vi "FiberSpectrograph_issueCommand_start.vi"(8 "error in (no error)":errorcluster, 11 "command_start_Ctl":T1) -> (0 "error out":errorcluster, 2 "function return":i32, 3 "command_start_Ctl out":T1)   [LabVIEW 2016, in "SALLV_FiberSpectrograph.lvlib"]
doc: "int FiberSpectrograph_shm_issueCommand_startLV(FiberSpectrograph_command_startLV *command_start_Ctl );"
uses:
  SALLV_FiberSpectrograph.lvlib
  DataTypes/command_start.ctl
  SALLV_FiberSpectrograph.so
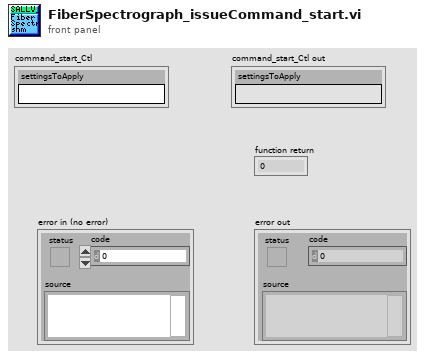
[diagram p1: front panel]
types:
  T1 = typedef "SALLV_FiberSpectrograph.lvlib/command_start.ctl" = cluster{"settingsToApply":string}
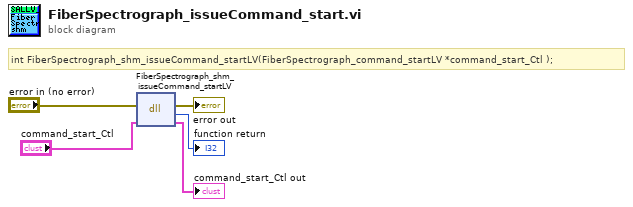
[diagram p0: block diagram]
diagram:
  # "int FiberSpectrograph_shm_issueCommand_startLV(FiberSpectrograph_command_startLV *command_start_Ctl );"
  n1 = dll-call lib="home/harini/tcs/sallv_FiberSpectrometer/SALLV_FiberSpectrograph.*" fn="FiberSpectrograph_shm_issueCommand_startLV"(error in="error in (no error)", "command_start_Ctl"="command_start_Ctl") -> (error out=→"error out":errorcluster, →"function return":i32, "command_start_Ctl"=→"command_start_Ctl out":T1)  [unwired: 2 in, 1 out]
